vi "Create File if Do Not Exist.vi"(8 "ErrorIn":errorcluster, 9 "FileName":string, 10 "FolderName":string, 11 "LogsClass In":refnum<class "LogsAbstract.lvclass">) -> (0 "ErrorOut":errorcluster, 1 "File Created?":bool, 3 "LogClass Out":refnum<class "LogsAbstract.lvclass">)   [LabVIEW 2019, in "LogsAbstract.lvlib" / "LogsAbstract.lvclass"]
uses:
  LogsAbstract.lvclass
  LogsAbstract.lvclass/LogsAbstract.ctl
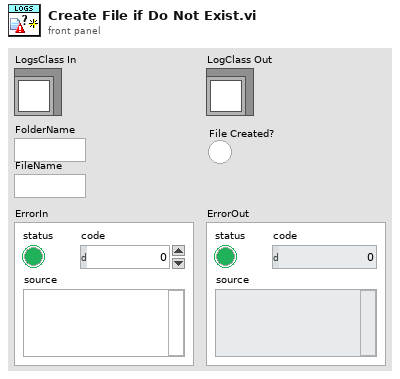
[diagram p1: front panel]
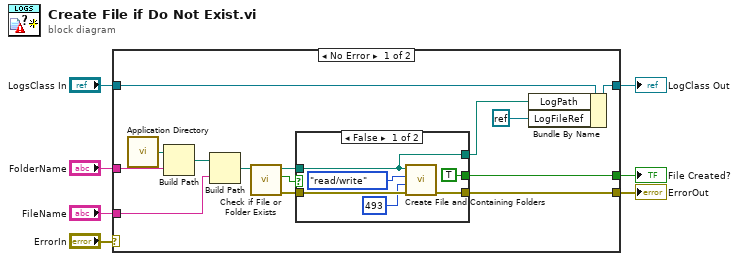
[diagram p0: block diagram]
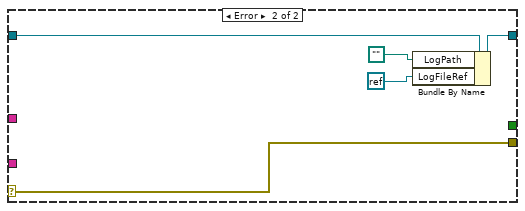
[diagram p3: hidden frame]
diagram:
  n1 = case shown="No Error" "ErrorIn" {
    selector: "ErrorIn" -> [_ w34]
    tunnel: "FolderName" -> [w20 _]
    tunnel: "FileName" -> [w19 _]
    tunnel: [w13 w34] -> w5
    tunnel: [w11 w32] -> w3
    tunnel: "LogsClass In" -> [w12 w33]
    tunnel: [w8 _] -> w1
    frame No Error {
      n2 = call <vilib>:"Application Directory.vi"() -> ("Application Directory"=w21:path)
      n3 = Build Path(base path=w21, name or relative path=w20) -> (appended path=w18:path)
      n4 = Build Path(base path=w18, name or relative path=w19) -> (appended path=w14:path)
      n5 = call <vilib>:"Check if File or Folder Exists.vi"("path"=w14) -> ("error out"=w17:errorcluster, "file or folder exists?"=w15:bool, "dup path"=w16:path)  [unwired: 8 in]
      n6 = case shown="False" w15 {
        tunnel: w16 -> [w25 w28]
        tunnel: w17 -> [w27 w29]
        tunnel: [w26 w29] -> w13
        tunnel: [w25 w28] -> w10
        tunnel: [TRUE _] -> w8
        frame False {
          n7 = call <vilib>:"Create File and Containing Folders.vi"("error in (no error)"=w27, "permissions"=i16 493, "access"=enum16{"read/write", "read-only", "write-only"}."read/write", "file path"=w25) -> ("error out"=w26:errorcluster)  [unwired: 6 in, 1 out]
        }
        frame True {
        }
      }
      n8 = Bundle By Name(cluster=w12, "LogPath"=w10, "LogFileRef"=refnum<k0> refnum) -> (w11:refnum<class "LogsAbstract.lvclass">)
    }
    frame Error {
      n9 = Bundle By Name(cluster=w33, "LogPath"=path "", "LogFileRef"=refnum<k0> refnum) -> (w32:refnum<class "LogsAbstract.lvclass">)
    }
  }
  "ErrorOut" <- w5
  "LogClass Out" <- w3
  "File Created?" <- w1
